vi "Signal Input.vi"(8 "error in (no error)":errorcluster, 9 "Gain":dbl=1.0 format="%_2p", 10 "Signal":dbl format="%_2p") -> (0 "error out":errorcluster)   [LabVIEW 2021, in "Haptic Prog Interface.lvlib"]
doc: "Inputs the signal of the pen for use in read or write mode, and allows for a configurable gain.\n\n<b>Signal:</b> Accepts a double, the value of the signal to be felt by the pen.\n\n<b>Gain:</b> Accepts a double, the value of the signal gain. Ultimately, gain * signal is felt by the pen."
uses:
  Haptic Prog Interface.lvlib
  Haptic-Programming-Interface/src/x64/Debug/Haptic Programming Interface.dll
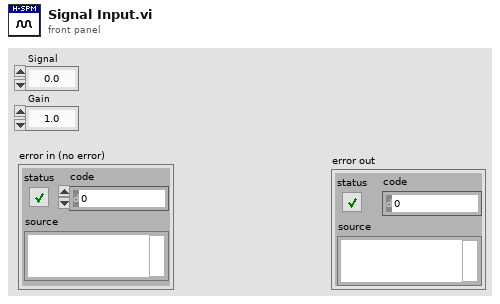
[diagram p1: front panel]
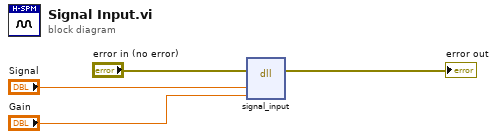
[diagram p0: block diagram]
diagram:
  n1 = dll-call lib="C:/Users/freem/Documents/GitHub/Haptic-Programming-Interface/src/x64/Debug/Haptic Programming Interface.dll" fn="signal_input"(error in="error in (no error)", "input_signal"="Signal", "input_gain"="Gain") -> (error out=→"error out":errorcluster)  [unwired: 5 in, 1 out]
